vi "ExerciceReservoir.vi"() -> ()   [LabVIEW 2018]
uses:
  ExerciceReservoir/Control 2.ctl
  ExerciceReservoir/Control 3.ctl
  ExerciceReservoir/Control 4.ctl
panel:
  in  "?":bool
  in  "Consigne":T1 max=1000 scale=0.0..1000.0
  in  "Débit":T2=1 min=1 max=10 scale=1.0..10.0
  out "Réservoir":T3 scale=0.0..1100.0
  # "[l/s]"
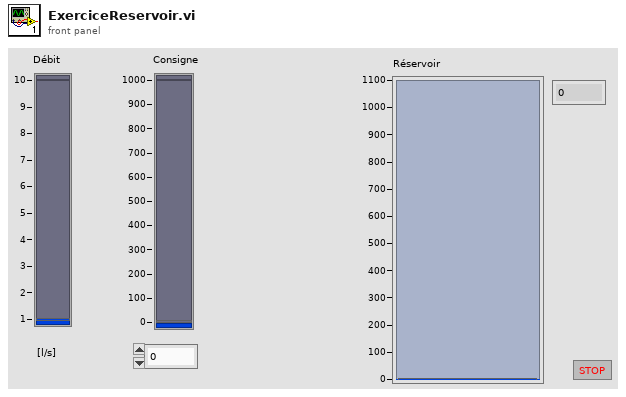
[diagram p1: front panel]
types:
  T1 = typedef "Control 2.ctl" = u16
  T2 = typedef "Control 3.ctl" = u8
  T3 = typedef "Control 4.ctl" = u16
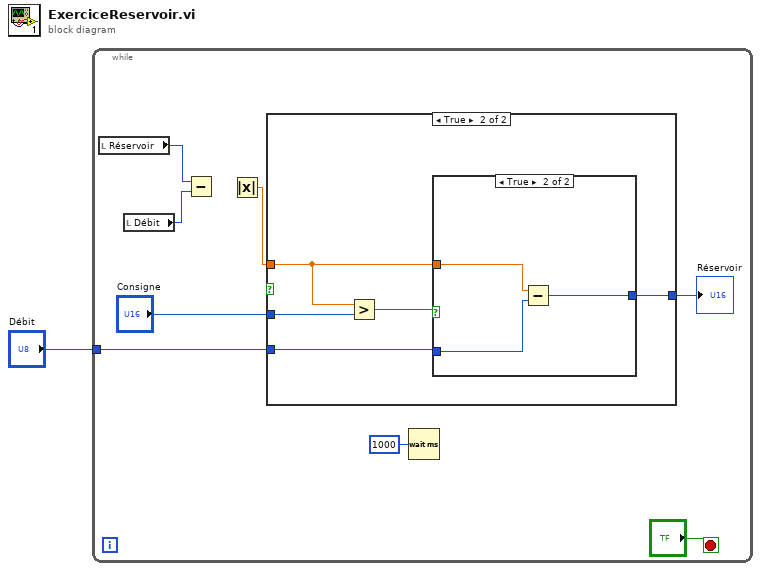
[diagram p0: block diagram]
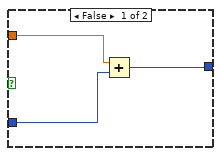
[diagram p3: hidden frame]
diagram:
  n1 = while {
    tunnel: "Débit" -> [w6]
    stop <- "?" stop-if-true
    n2 = local read "Réservoir"() -> (w4:T3)
    n3 = local read "Débit"() -> (w3:T2)
    n4 = Subtract(x=w4, y=w3) -> ()  [unwired: 1 out]
    n5 = Absolute Value() -> (abs(x)=w2:dbl)  [unwired: 1 in]
    n6 = case shown="True" {
      selector: _ -> [_ _]
      tunnel: [_ w13] -> w7
      tunnel: w6 -> [_ w12]
      tunnel: w2 -> [_ w11]
      tunnel: "Consigne" -> [_ w10]
      frame False {
      }
      frame True {
        n7 = Greater?(x=w11, y=w10) -> (0:w14:bool)
        n8 = case shown="True" w14 {
          tunnel: w11 -> [w17 w19]
          tunnel: [w16 w20] -> w13
          tunnel: w12 -> [w15 w18]
          frame False {
            n9 = Add(x=w17, y=w15) -> (x+y=w16:T2)
          }
          frame True {
            n10 = Subtract(x=w19, y=w18) -> (x-y=w20:T2)
          }
        }
      }
    }
    "Réservoir" <- w7
    n11 = Wait (ms)(milliseconds to wait=u32 1000) -> ()  [unwired: 1 out]
  }
